vi "SR430.byte array to waveform.vi"(7 "byteArray out":T1) -> (8 "Waveform":waveform(dbl))   [LabVIEW 2014, in "SR430.lvlib"]
doc: "Converts an array of bytes to a waveform according to a convention (D:1, D:1, D:N)"
uses:
  SR430.lvlib
  CS_Core/CSSystem/CoreDefs/CoreDefs.rawDataType.ctl
  CS_Core/CSSystem/CoreLib/CoreLib.byte array 2 double.vi
  CS_Core/CSSystem/CoreLib/CoreLib.byte array 2 double array.vi
  CS_Core/CSSystem/CoreLib/CoreLib.lvlib
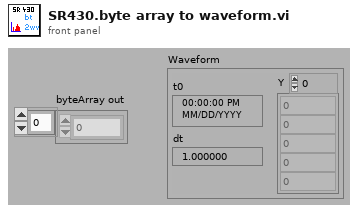
[diagram p1: front panel]
types:
  T1 = typedef "CoreDefs.rawDataType.ctl" = i8[]
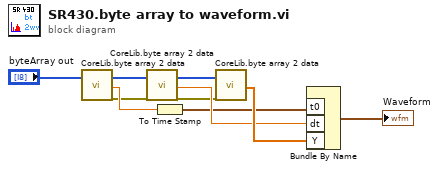
[diagram p0: block diagram]
diagram:
  n1 = call-poly "CoreLib.byte array 2 data.vi"("byteArray"="byteArray out") -> ("byteArray out"=w9:T1, "d64"=w4:dbl, "error out"=w2:errorcluster)  [unwired: 16 in]
  n2 = call-poly "CoreLib.byte array 2 data.vi"("byteArray"=w9, "error in (no error)"=w2) -> ("byteArray out"=w8:T1, "d64"=w5:dbl, "error out"=w1:errorcluster)  [unwired: 15 in]
  n3 = To Time Stamp(1:w4) -> (0:w3:timestamp)
  n4 = call-poly "CoreLib.byte array 2 data.vi"("byteArray"=w8, "error in (no error)"=w1) -> ("[d64]"=w6:dbl[])  [unwired: 15 in, 2 out]
  n5 = Bundle By Name("t0"=w3, "dt"=w5, "Y"=w6) -> (→"Waveform":waveform(dbl))  [unwired: 1 in]
